vi "Get Data.vi"(8 "error in":errorcluster, 11 "GUI in":refnum<class "GUI.lvclass">) -> (0 "error out":errorcluster, 2 "Data":refnum<class "Data.lvclass">, 3 "GUI out":refnum<class "GUI.lvclass">)   [LabVIEW 2012, in "GUI.lvclass"]
uses:
  GUI.lvclass
  Data/Data.lvclass
  GUI.lvclass/GUI.ctl
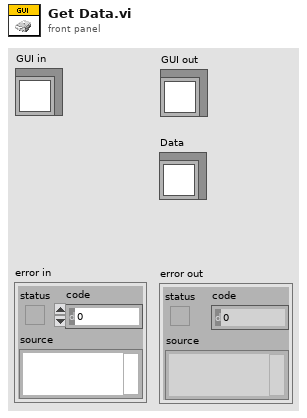
[diagram p1: front panel]
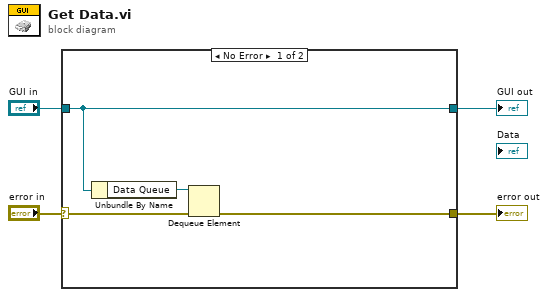
[diagram p0: block diagram]
diagram:
  n1 = case shown="No Error" "error in" {
    selector: "error in" -> [w7 w10]
    tunnel: [w5 w10] -> w3
    tunnel: [w6 w9] -> w1
    tunnel: "GUI in" -> [w6 w9]
    frame No Error {
      n2 = Unbundle By Name(w6) -> ("Data Queue"=w8:refnum<queue>)
      n3 = Dequeue Element(queue=w8, error in (no error)=w7) -> (error out=w5:errorcluster)  [unwired: 1 in, 3 out]
    }
    frame Error {
    }
  }
  "error out" <- w3
  "GUI out" <- w1
